vi "create_motor_scan_files.vi"(8 "error in (no error)":errorcluster, 11 "base path":path) -> (0 "error out":errorcluster, 1 "New Folder Created?":bool, 2 "Ref Num Array":refnum<file>[](array[refnum]), 3 "Save Files Array":path[](array[path]), 4 "Scan Number":i32)   [LabVIEW 2018]
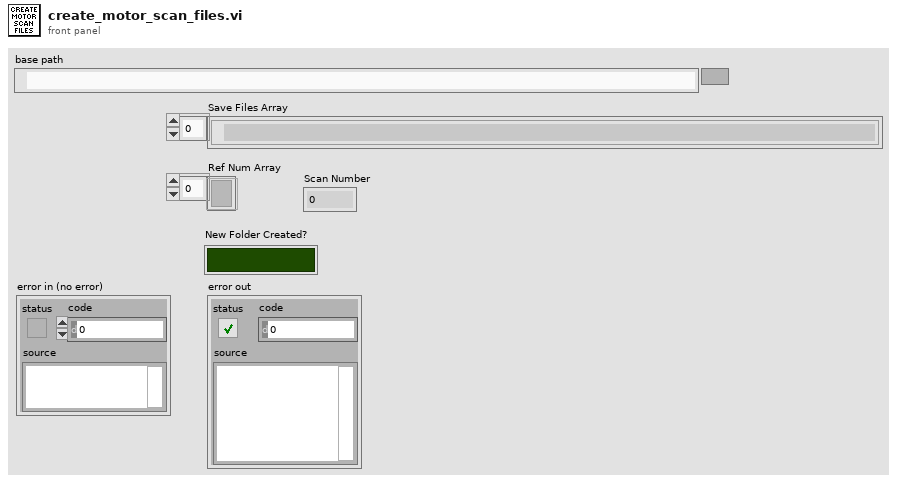
[diagram p1: front panel]
types:
  T1 = enum16{"open", "replace", "create", "open or create", "replace or create", "replace or create with confirmation"}
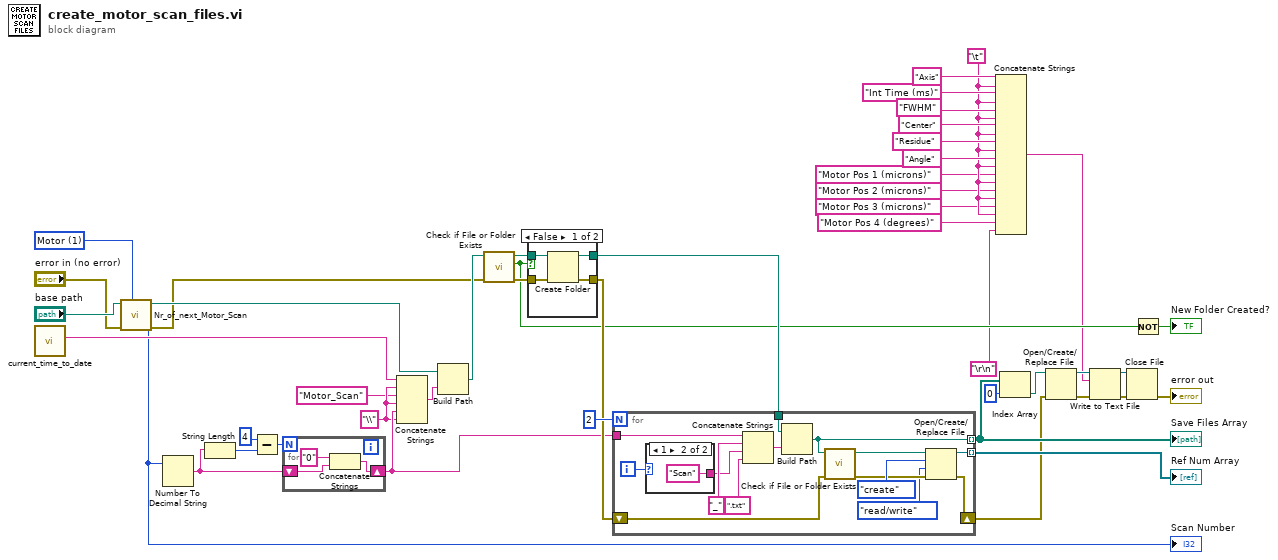
[diagram p0: block diagram]
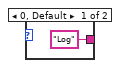
[diagram p3: hidden frame]
diagram:
  w7 = u16 1 items=["Energy / Time", "Motor", "TDC", "Keithley"] ("Scan Type")
  w6 = "\t"
  w32 = "\\" ("string")
  n1 = call "current_time_to_date.vi"() -> ("yyyy-mm-dd"=w41:string)  [unwired: 10 in, 1 out]
  n2 = call "Nr_of_next_Motor_Scan.vi"("Scan Type"=w7, "error in (no error)"="error in (no error)", "base path"="base path") -> ("error out"=w26:errorcluster, "scan nr"=w15:i32, "path out"=w28:path)  [unwired: 6 in]
  "Scan Number" <- w15
  n3 = Number To Decimal String(number=w15) -> (decimal integer string=w43:string)  [unwired: 1 in]
  n4 = String Length(string=w43) -> (length=w46:i32)
  n5 = Subtract(x=4, y=w46) -> (x-y=w44:i32)
  n6 = for {
    N: w44 -> [_]
    shift-right: [w47] -> w33
    shift-left: w43 -> [w48]
    n7 = Concatenate Strings("0", w48) -> (w47:string)
  }
  n8 = Concatenate Strings(w41, w32, "Motor_Scan" ("string"), w32, w33, w32) -> (w36:string)
  n9 = Build Path(base path=w28, name or relative path=w36) -> (appended path=w40:path)
  n10 = call <vilib>:"Check if File or Folder Exists.vi"("error in (no error)"=w26, "path"=w40) -> ("error out"=w37:errorcluster, "file or folder exists?"=w31:bool, "dup path"=w39:path)  [unwired: 7 in]
  n11 = case shown="False" w31 {
    tunnel: w39 -> [w53 w55]
    tunnel: [w52 w55] -> w38
    tunnel: w37 -> [w51 w54]
    tunnel: [w50 w54] -> w35
    frame False {
      n12 = Create Folder(path (use dialog)=w53, error in=w51) -> (created path=w52:path, error out=w50:errorcluster)  [unwired: 1 in, 1 out]
    }
    frame True {
    }
  }
  n13 = for {
    N: 2 -> [_]
    tunnel: w33 -> [w69]
    tunnel: w38 -> [w68]
    tunnel: [w63] -> w25 mode=indexing
    shift-right: [w58] -> w18
    shift-left: w35 -> [w59]
    tunnel: [w56] -> w34 mode=indexing
    i -> [w65]
    n14 = case shown="1" w65 {
      tunnel: ["Log" ("string") "Scan" ("string")] -> w64
      frame 0, Default {
      }
      frame 1 {
      }
    }
    n15 = Concatenate Strings(w69, "_" ("string"), w64, ".txt" ("string")) -> (w70:string)
    n16 = Build Path(base path=w68, name or relative path=w70) -> (appended path=w63:path)
    n17 = call <vilib>:"Check if File or Folder Exists.vi"("error in (no error)"=w59, "path"=w63) -> ("error out"=w60:errorcluster, "dup path"=w62:path)  [unwired: 7 in, 1 out]
    n18 = Open/Create/Replace File(file path (use dialog)=w62, error in=w60, operation (0:open)=T1."create", access (0:read/write)=enum16{"read/write", "read-only", "write-only"}."read/write") -> (refnum out=w56:refnum<file>, error out=w58:errorcluster)  [unwired: 2 in, 1 out]
  }
  "Save Files Array" <- w25
  "Ref Num Array" <- w34
  n19 = Concatenate Strings("Axis" ("text"), w6, "Int Time (ms)" ("text"), w6, "FWHM" ("text"), w6, "Center" ("text"), w6, "Residue" ("text"), w6, "Angle" ("text"), w6, "Motor Pos 1 (microns)" ("text"), w6, "Motor Pos 2 (microns)" ("text"), w6, "Motor Pos 3 (microns)" ("text"), w6, "Motor Pos 4 (degrees)" ("text"), "\r\n") -> (w16:string)
  n20 = Index Array(array=w25, index=0) -> (element=w23:path)
  n21 = Open/Create/Replace File(file path (use dialog)=w23, error in=w18) -> (refnum out=w21:refnum<file>, error out=w22:errorcluster)  [unwired: 4 in, 1 out]
  n22 = Write to Text File(file (use dialog)=w21, text=w16, error in=w22) -> (refnum out=w20:refnum<file>, error out=w19:errorcluster)  [unwired: 1 in, 1 out]
  n23 = Close File(refnum=w20, error in=w19) -> (error out=→"error out":errorcluster)  [unwired: 1 out]
  n24 = Not(x=w31) -> (.not. x?=→"New Folder Created?":bool)
